vi "Write Spreadsheet.vi"(8 "error in (no error)":errorcluster, 11 "Excel XML in":refnum<class "Excel XML.lvclass">) -> (0 "error out":errorcluster, 3 "Excel XML out":refnum<class "Excel XML.lvclass">)   [LabVIEW 2013, in "Excel XML.lvclass"]
uses:
  Excel XML.lvclass
  Spreadsheet.lvclass
  Excel XML.lvclass/Excel XML.ctl
  C:/PhaeronGit/LVNPOI/Resources/NPOI 2.1.1 dotnet4/NPOI.OOXML.dll
  Resources/NPOI 2.1.1 dotnet4/NPOI.OOXML.dll
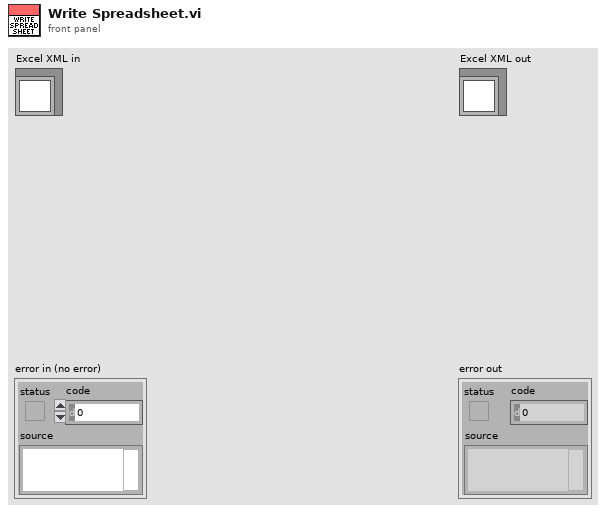
[diagram p1: front panel]
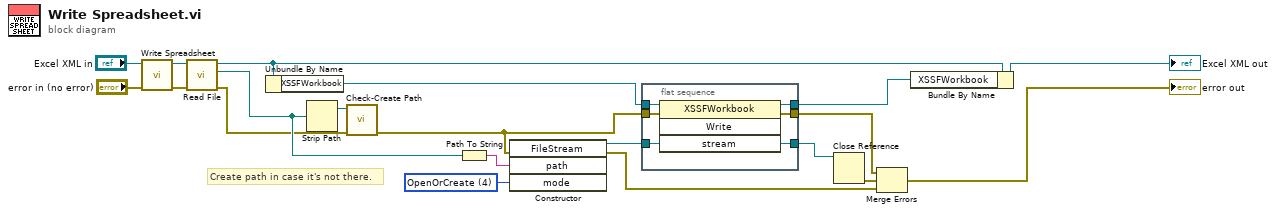
[diagram p0: block diagram]
diagram:
  w14 = 4 items=["CreateNew"=1, "Create"=2, "Open"=3, "OpenOrCreate"=4, "Truncate"=5, "Append"=6] ("mode")
  # "Create path in case it's not there."
  n1 = call-parent "Write Spreadsheet.vi"("error in (no error)"="error in (no error)", "Spreadsheet in"="Excel XML in") -> ("error out"=w6:errorcluster, "Spreadsheet out"=w5:refnum<class "Excel XML.lvclass">)  [unwired: 8 in]
  n2 = call-dynamic "Read File.vi"("error in (no error)"=w6, "Spreadsheet in"=w5) -> ("error out"=w16:errorcluster, "File"=w19:path, "Spreadsheet out"=w17:refnum<class "Excel XML.lvclass">)  [unwired: 7 in]
  n3 = Unbundle By Name(w17) -> ("XSSFWorkbook"=w18:refnum<k24>)
  n4 = Strip Path(path=w19) -> (stripped path=w7:path)  [unwired: 1 out]
  n5 = call <vilib>:"Check-Create Path.vi"("error in"=w16, "Path"=w7) -> ("error out"=w8:errorcluster)  [unwired: 8 in, 1 out]
  n6 = Path To String(path=w19) -> (string=w15:string)
  n7 = constructor class="FileStream"(error in=w8, "path"=w15, "mode"=w14) -> (reference out=w13:refnum<k24>, error out=w9:errorcluster)  [unwired: 2 in, 3 out]
  n8 = flat-sequence {
    tunnel: w18 -> [w25]
    tunnel: [w24] -> w20
    tunnel: w8 -> [w23]
    tunnel: w13 -> [w21]
    tunnel: [w22] -> w12
    tunnel: [w21] -> w10
    frame #0 {
      n9 = invoke class="XSSFWorkbook" method="Write"(reference=w25, error in=w23, "stream"=w21) -> (reference out=w24:refnum<k24>, error out=w22:errorcluster)  [unwired: 1 in, 2 out]
    }
  }
  n10 = Close Reference(reference=w10) -> (error out=w11:errorcluster)  [unwired: 1 in]
  n11 = Merge Errors(w12, w11, w9) -> (→"error out":errorcluster)
  n12 = Bundle By Name(cluster=w17, "XSSFWorkbook"=w20) -> (→"Excel XML out":refnum<class "Excel XML.lvclass">)
